vi "LVClass_HasoSlopes dtor.vi"(0 "HasoSlopes in":refnum<class "HasoSlopes.lvclass">, 11 "error in (no error)":errorcluster) -> (4 "HasoSlopes out":refnum<class "HasoSlopes.lvclass">, 15 "error out":errorcluster)   [LabVIEW 2020, in "HasoSlopes.lvclass"]
doc: "HasoSlopes destructor.\n\n--------------------------------------------------------------------------------\n\n<B>HasoSlopesIn </B> : HasoSlopes object.\n<B>HasoSlopesOut </B> : HasoSlopes object.\n<B>ErrorIn </B> : Error\n<B>ErrorOut </B> : Error\n\n--------------------------------------------------------------------------------"
uses:
  HasoSlopes.lvclass
  HasoSlopes.lvclass/HasoSlopes.ctl
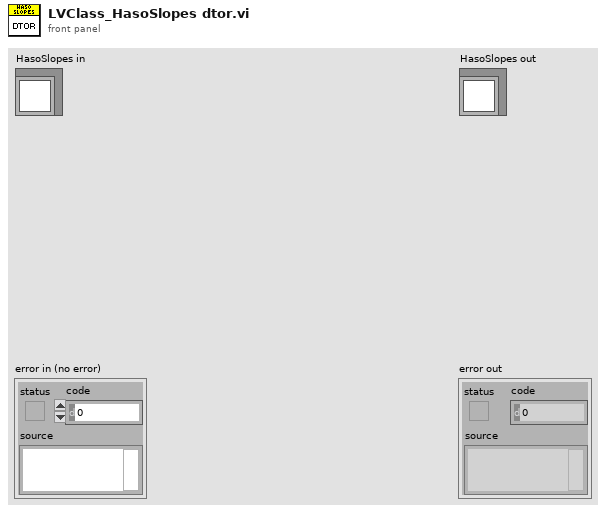
[diagram p1: front panel]
types:
  T1 = typedef "Handle creation.ctl" = enum16{"By ctor", "By write function"}
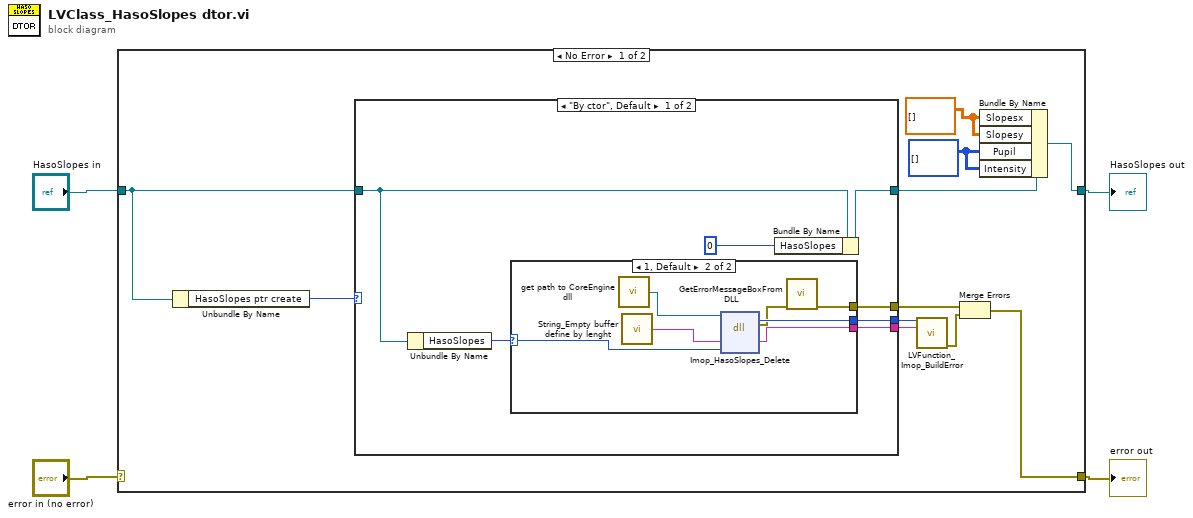
[diagram p0: block diagram]
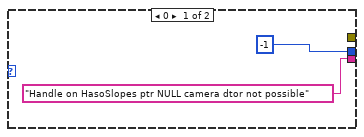
[diagram p2: hidden frame]
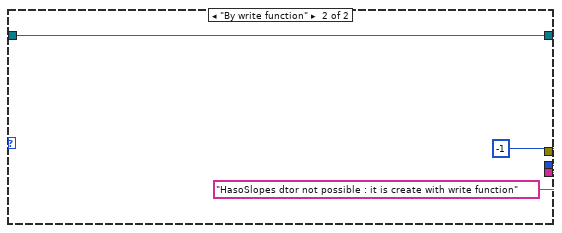
[diagram p3: hidden frame]
diagram:
  n1 = case shown="No Error" "error in (no error)" {
    selector: "error in (no error)" -> [_ w36]
    tunnel: [w9 w36] -> w3
    tunnel: [w7 w35] -> w2
    tunnel: "HasoSlopes in" -> [w13 w35]
    frame No Error {
      w5 = i32[][] [] ("Pupil")
      w6 = sgl[][] [] ("Slopesx")
      n2 = Unbundle By Name(w13) -> ("HasoSlopes ptr create"=w12:T1)
      n3 = case shown="\"By ctor\", Default" w12 {
        tunnel: w13 -> [w18 w34]
        tunnel: [w22 w34] -> w8
        tunnel: [w20 -1] -> w15
        tunnel: [w19 "HasoSlopes dtor not possible : it is create with write function" ("message")] -> w14
        tunnel: [w16 _] -> w11
        frame "By ctor", Default {
          n4 = Unbundle By Name(w18) -> ("HasoSlopes"=w17:i32)
          n5 = case shown="1, Default" w17 {
            selector: w17 -> [_ w28]
            tunnel: ["Handle on HasoSlopes ptr NULL camera dtor not possible" ("message") w30] -> w19
            tunnel: [-1 w29] -> w20
            tunnel: [_ w25] -> w16
            frame 0 {
            }
            frame 1, Default {
              n6 = call "get path to CoreEngine dll.vi"() -> ("path to c_interface_vc100.dll"=w27:path)  [unwired: 12 in, 3 out]
              n7 = call "String_Empty buffer define by lenght.vi"() -> ("Empty buffer"=w31:string)  [unwired: 1 in]
              n8 = dll-call lib="D:/soft/HASO_v3/SVN_trunk/ImOpCoreEngine4_LV2011/DLLs/c_interface_vc100.dll" fn="Imop_HasoSlopes_Delete"(path in=w27, "message"=w31, "objet"=w28) -> (error out=w26:errorcluster, "return type"=w29:i32, "message"=w30:string)  [unwired: 3 in, 1 out]
              n9 = call "GetErrorMessageBoxFromDLL.vi"("error IN"=w26) -> ("error OUT"=w25:errorcluster)  [unwired: 10 in]
            }
          }
          n10 = Bundle By Name(cluster=w18, "HasoSlopes"=u32 0) -> (w22:refnum<class "HasoSlopes.lvclass">)
        }
        frame "By write function" {
        }
      }
      n11 = call "LVFunction_Imop_BuildError.vi"("code"=w15, "String to Prepend to source (\"\")"=w14) -> ("error out"=w10:errorcluster)  [unwired: 13 in]
      n12 = Merge Errors(w11, w10) -> (w9:errorcluster)
      n13 = Bundle By Name(cluster=w8, "Slopesx"=w6, "Slopesy"=w6, "Pupil"=w5, "Intensity"=w5) -> (w7:refnum<class "HasoSlopes.lvclass">)
    }
    frame Error {
    }
  }
  "error out" <- w3
  "HasoSlopes out" <- w2
